vi "Auton - Center Gear No Vision.vi"(11 "Auton States":T1) -> ()   [LabVIEW 2016]
uses:
  Auton - Center Gear No Vision States.ctl
panel:
  in  "Tolerance":dbl=2.0 format="%#_13g"
  out "Current State":T1
  in  "Back Away SP":dbl
  in  "Drive Forward SP":dbl=72.0
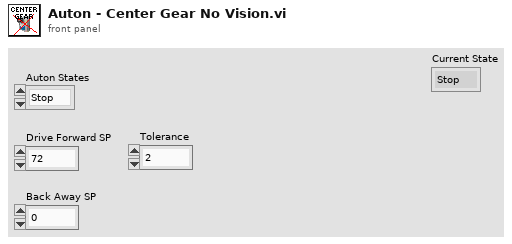
[diagram p1: front panel]
types:
  T1 = typedef "Auton - Center Gear No Vision States.ctl" = enum16{"Stop", "Reset Encoders", "Drive to Peg", "Eject Gear", "Back Away"}
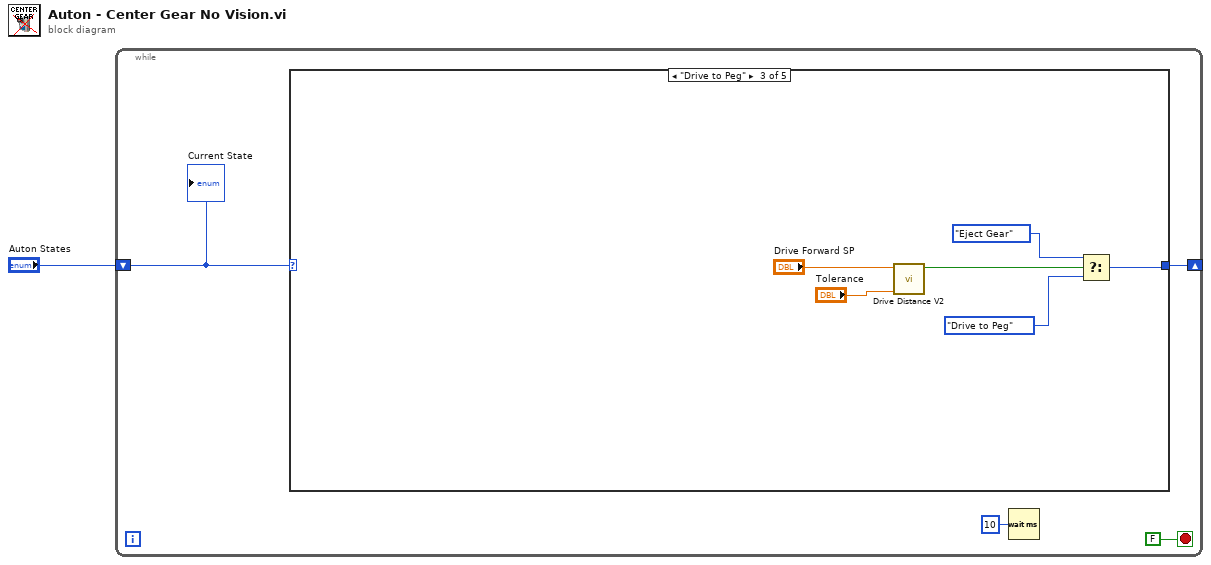
[diagram p0: block diagram]
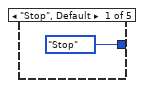
[diagram p2: hidden frame]
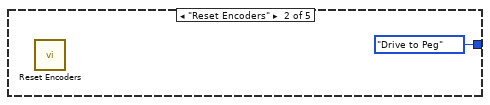
[diagram p3: hidden frame]
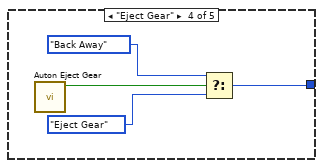
[diagram p4: hidden frame]
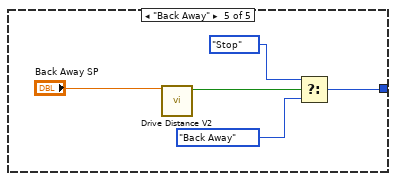
[diagram p5: hidden frame]
diagram:
  n1 = while {
    shift-right: [w2] -> _
    shift-left: "Auton States" -> [w3]
    stop <- FALSE stop-if-true
    n2 = case shown="\"Drive to Peg\"" w3 {
      tunnel: [Auton_-_Center_Gear_No_Vision_States."Stop" ("Auton States") Auton_-_Center_Gear_No_Vision_States."Drive to Peg" ("Auton States") w13 w17 w22] -> w2
      frame "Stop", Default {
      }
      frame "Reset Encoders" {
        n3 = call "Reset Encoders.vi"() -> ()  [unwired: 11 in, 1 out]
      }
      frame "Drive to Peg" {
        n4 = call "Drive Distance V2.vi"("Tolerance"="Tolerance", "Distance Set Point"="Drive Forward SP") -> ("Done?"=w10:bool)  [unwired: 9 in]
        n5 = Select(t=Auton_-_Center_Gear_No_Vision_States."Eject Gear" ("Auton States"), s=w10, f=Auton_-_Center_Gear_No_Vision_States."Drive to Peg" ("Auton States")) -> (s? t:f=w13:T1)
      }
      frame "Eject Gear" {
        n6 = call "Auton Eject Gear.vi"() -> ("Done?"=w16:bool)  [unwired: 11 in]
        n7 = Select(t=Auton_-_Center_Gear_No_Vision_States."Back Away" ("Auton States"), s=w16, f=Auton_-_Center_Gear_No_Vision_States."Eject Gear" ("Auton States")) -> (s? t:f=w17:T1)
      }
      frame "Back Away" {
        n8 = call "Drive Distance V2.vi"("Distance Set Point"="Back Away SP") -> ("Done?"=w21:bool)  [unwired: 10 in]
        n9 = Select(t=Auton_-_Center_Gear_No_Vision_States."Stop" ("Auton States"), s=w21, f=Auton_-_Center_Gear_No_Vision_States."Back Away" ("Auton States")) -> (s? t:f=w22:T1)
      }
    }
    n10 = Wait (ms)(milliseconds to wait=u32 10) -> ()  [unwired: 1 out]
    "Current State" <- w3
  }
